vi "Enable Channel Output.vi"(8 "error in (no error)":errorcluster, 9 "Channel (1: 1)":u16(ring)=1 items=["1"=1, "2"=2], 10 "Enable Output (T: Enable)":bool=TRUE, 11 "VISA resource name":refnum<visa-resource-name>) -> (0 "error out":errorcluster, 3 "VISA resource name out":refnum<visa-resource-name>)   [LabVIEW 2019, in "Agilent 3352X Series.lvlib"]
doc: "Enables or disables the front panel output connector."
uses:
  Agilent 3352X Series.lvlib
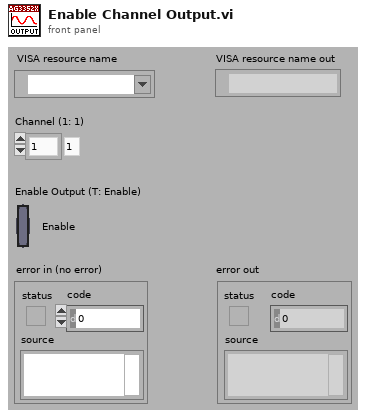
[diagram p1: front panel]
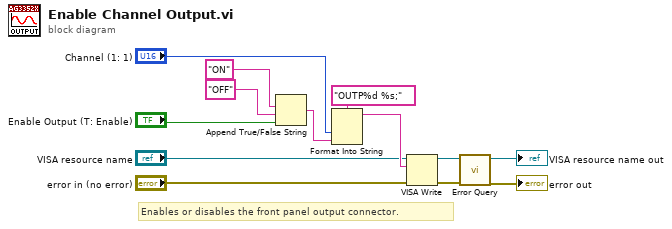
[diagram p0: block diagram]
diagram:
  # "Enables or disables the front panel output connector."
  n1 = Append True/False String(1:"Enable Output (T: Enable)", 2:"OFF", 3:"ON") -> (0:w8:string)  [unwired: 1 out]
  n2 = Format Into String(format string="OUTP%d %s;", "Channel (1: 1)", w8) -> (resulting string=w7:string)  [unwired: 2 in, 1 out]
  n3 = VISA Write(VISA resource name="VISA resource name", write buffer=w7, error in (no error)="error in (no error)") -> (VISA resource name out=w4:refnum<visa-resource-name>, error out=w3:errorcluster)  [unwired: 1 out]
  n4 = call "Error Query.vi"("error in (no error)"=w3, "VISA resource name"=w4) -> ("error out"=→"error out":errorcluster, "VISA resource name out"=→"VISA resource name out":refnum<visa-resource-name>)  [unwired: 8 out]
